vi "Get Last Log Part.vi"(7 "Logger Output":T1, 8 "error in (no error)":errorcluster, 9 "Filetype":string, 10 "Filename":string, 11 "Root path in":path) -> (0 "error out":errorcluster, 2 "File write position":i64, 3 "File to Write in ref":refnum<file>)   [LabVIEW 2016, in "Global_logger.lvlib"]
uses:
  Global_logger.lvlib
  Logger Output.ctl
  Levels.ctl
  Level Meaning.ctl
  Sorting.ctl
  Logger Type.ctl
  Log Fields.ctl
  <userlib>/_OpenG.lib/file/file.llb/File Exists - Scalar__ogtk.vi
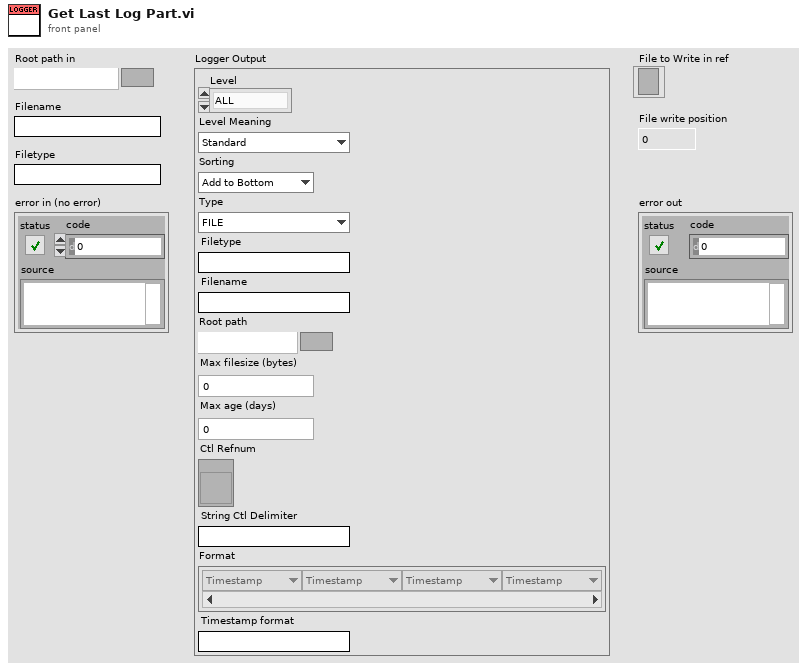
[diagram p1: front panel]
types:
  T1 = typedef "Global_logger.lvlib/Logger Output.ctl" = cluster{"Level":T2, "Level Meaning":T3, "Sorting":T4, "Type":T5, "Filetype":string, "Filename":string, "Root path":path, "Max filesize (bytes)":i32, "Max age (days)":i32, "Ctl Refnum":refnum<vi>, "String Ctl Delimiter":string, "Format":T6[], "Timestamp format":string}
  T2 = typedef "Global_logger.lvlib/Levels.ctl" = enum16{"ALL", "TRACE", "DEBUG", "INFO", "WARN", "ERROR", "FATAL", "OFF"}
  T3 = typedef "Global_logger.lvlib/Level Meaning.ctl" = enum16{"Standard", "Positive", "Exact"}
  T4 = typedef "Global_logger.lvlib/Sorting.ctl" = enum16{"Add to Bottom", "Add to Top"}
  T5 = typedef "Global_logger.lvlib/Logger Type.ctl" = enum16{"FILE", "UI"}
  T6 = typedef "Global_logger.lvlib/Log Fields.ctl" = enum16{"Timestamp", "Level", "Message", "Source VI", "Source App", "Logger Name"}
  T7 = enum16{"open", "replace", "create", "open or create", "replace or create", "replace or create with confirmation"}
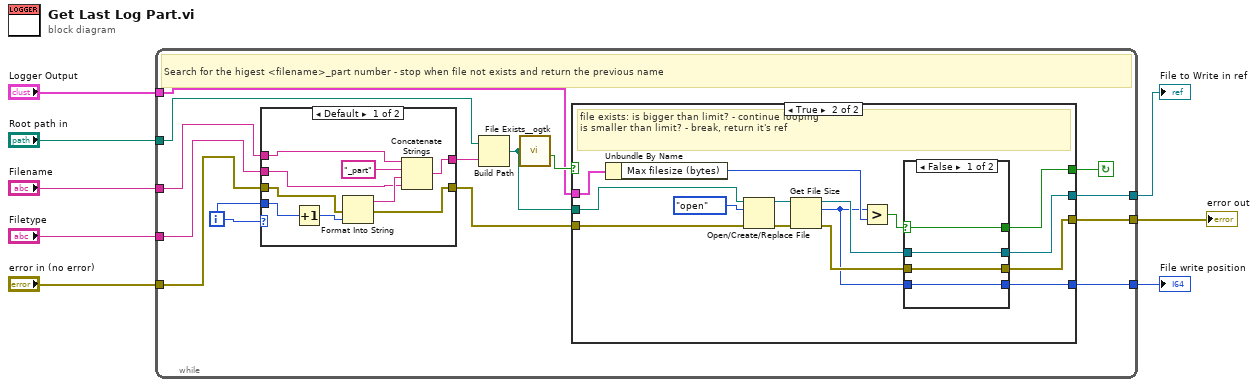
[diagram p0: block diagram]
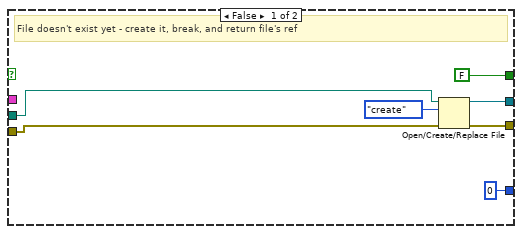
[diagram p2: hidden frame]
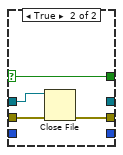
[diagram p3: hidden frame]
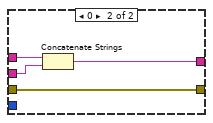
[diagram p4: hidden frame]
diagram:
  n1 = while {
    tunnel: [w12] -> w6
    tunnel: "error in (no error)" -> [w18]
    tunnel: "Filename" -> [w21]
    tunnel: "Filetype" -> [w20]
    tunnel: "Root path in" -> [w22]
    tunnel: "Logger Output" -> [w14]
    tunnel: [w10] -> w2
    tunnel: [w9] -> w1
    i -> [w19]
    stop <- w11 continue-if-true
    # "Search for the higest <filename>_part number - stop when file not exists and return the previous name"
    n2 = case shown="Default" w19 {
      tunnel: w21 -> [w61 w65]
      tunnel: w20 -> [w53 w64]
      tunnel: w19 -> [w59 _]
      tunnel: w18 -> [w57 w62]
      tunnel: [w56 w62] -> w13
      tunnel: [w54 w63] -> w17
      frame Default {
        n3 = Increment(x=w59) -> (x+1=w58:i32)
        n4 = Format Into String(error in=w57, w58) -> (resulting string=w55:string, error out=w56:errorcluster)  [unwired: 2 in]
        n5 = Concatenate Strings(w61, "_part" ("string"), w55, w53) -> (w54:string)
      }
      frame 0 {
        n6 = Concatenate Strings(w65, w64) -> (w63:string)
      }
    }
    n7 = Build Path(base path=w22, name or relative path=w17) -> (appended path=w15:path)
    n8 = call-poly <userlib>:"File Exists__ogtk.vi"("file path"=w15) -> ("exists"=w16:bool)  [unwired: 6 in, 1 out]
    n9 = case shown="True" w16 {
      tunnel: w13 -> [w29 w42]
      tunnel: [w27 w32] -> w10
      tunnel: [w26 w36] -> w12
      tunnel: w15 -> [w25 w40]
      tunnel: w14 -> [_ w39]
      tunnel: [FALSE w33] -> w11
      tunnel: [i64 0 ("size (in bytes)") w31] -> w9
      frame False {
        # "File doesn't exist yet - create it, break, and return file's ref"
        n10 = Open/Create/Replace File(file path (use dialog)=w25, error in=w29, operation (0:open)=T7."create") -> (refnum out=w27:refnum<file>, error out=w26:errorcluster)  [unwired: 3 in, 1 out]
      }
      frame True {
        # "file exists: is bigger than limit? - continue looping\nis smaller than limit? - break, return it's ref"
        n11 = Unbundle By Name(w39) -> ("Max filesize (bytes)"=w38:i32)
        n12 = Open/Create/Replace File(file path (use dialog)=w40, error in=w42, operation (0:open)=T7."open") -> (refnum out=w44:refnum<file>, error out=w41:errorcluster)  [unwired: 3 in, 1 out]
        n13 = Get File Size(file=w44, error in=w41) -> (refnum out=w35:refnum<file>, size (in bytes)=w30:i64, 0:w37:errorcluster)
        n14 = Greater?(x=w30, y=w38) -> (0:w34:bool)
        n15 = case shown="False" w34 {
          selector: w34 -> [w47 w49]
          tunnel: w37 -> [w48 w52]
          tunnel: [w48 w51] -> w36
          tunnel: w35 -> [w46 w50]
          tunnel: [w47 w49] -> w33
          tunnel: [w46 _] -> w32
          tunnel: [w45 _] -> w31
          tunnel: w30 -> [w45 _]
          frame False {
          }
          frame True {
            n16 = Close File(refnum=w50, error in=w52) -> (error out=w51:errorcluster)  [unwired: 1 out]
          }
        }
      }
    }
  }
  "error out" <- w6
  "File to Write in ref" <- w2
  "File write position" <- w1
